vi "Felder Farben zuweisen.vi"(8 "Fehler":bool, 9 "Aktiv":bool, 11 "Element":refnum<vi>) -> ()   [LabVIEW 2020, in "Status Analysatoren.lvlib"]
uses:
  Status Analysatoren.lvlib
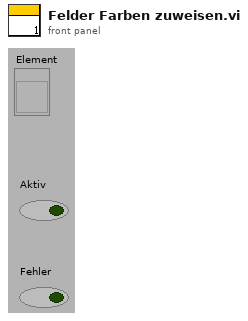
[diagram p1: front panel]
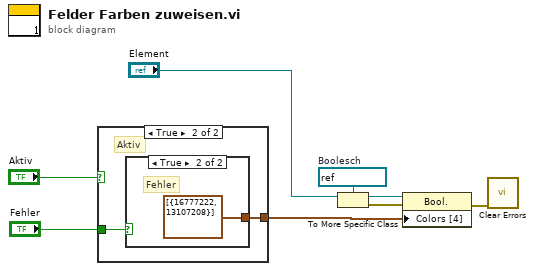
[diagram p0: block diagram]
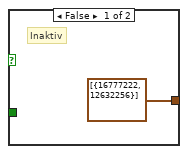
[diagram p2: hidden frame]
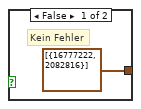
[diagram p3: hidden frame]
diagram:
  w8 = refnum<vi> refnum  # Boolesch
  n1 = case shown="True" "Aktiv" {
    tunnel: "Fehler" -> [_ w11]
    tunnel: [cluster{"Farbfeld":u32, "Farbfeld 2":u32}[] [{"Farbfeld"=16777222, "Farbfeld 2"=12632256}] ("Array") w10] -> w6
    frame False {
      # "Inaktiv"
    }
    frame True {
      # "Aktiv"
      n2 = case shown="True" w11 {
        tunnel: [cluster{"Farbfeld":u32, "Farbfeld 2":u32}[] [{"Farbfeld"=16777222, "Farbfeld 2"=2082816}] ("Array") cluster{"Farbfeld":u32, "Farbfeld 2":u32}[] [{"Farbfeld"=16777222, "Farbfeld 2"=13107208}] ("Array")] -> w10
        frame False {
          # "Kein Fehler"
        }
        frame True {
          # "Fehler"
        }
      }
    }
  }
  n3 = To More Specific Class(target class=w8, reference="Element") -> (specific class reference=w7:refnum<vi>, error out=w2:errorcluster)  [unwired: 1 in]
  n4 = property class="Bool."(reference=w7, error in=w2, "Colors [4]"=w6) -> (error out=w1:errorcluster)  [unwired: 1 out]
  n5 = call <vilib>:"Clear Errors.vi"("error in (no error)"=w1) -> ()  [unwired: 5 in, 2 out]
